vi "SEQ Destroy.vi"(8 "error in (no error)":errorcluster, 10 "wait for activity?":bool, 11 "Data Refnum":T1) -> (0 "error out":errorcluster, 3 "Final Data":T2)   [LabVIEW 2009]
doc: "This is a template VI for the SEQ Destroy functionality.\n\nAAL 9/09"
uses:
  Controls/SEQ Data.ctl
  Controls/SEQ DataRef.ctl
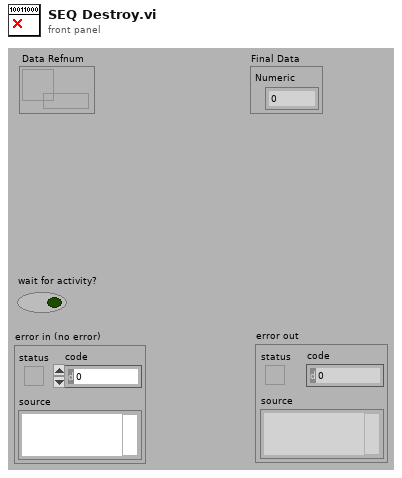
[diagram p1: front panel]
types:
  T1 = typedef "SEQ DataRef.ctl" = refnum<queue>
  T2 = typedef "SEQ Data.ctl" = cluster{"Numeric":dbl}
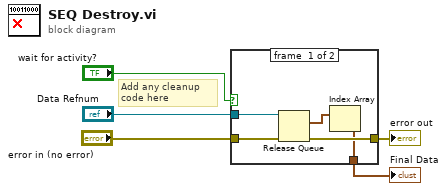
[diagram p0: block diagram]
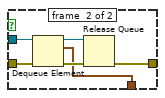
[diagram p2: hidden frame]
diagram:
  # "Add any cleanup\ncode here"
  n1 = case shown="False" "wait for activity?" {
    tunnel: "error in (no error)" -> [w8 w16]
    tunnel: "Data Refnum" -> [w7 w15]
    tunnel: [w10 w12] -> w3
    tunnel: [w6 w11] -> w2
    frame #0 {
      n2 = Release Queue(queue=w7, error in (no error)=w8) -> (remaining elements=w9:T2[], error out=w10:errorcluster)  [unwired: 2 out]
      n3 = Index Array(array=w9) -> (element=w6:T2)  [unwired: 1 in]
    }
    frame #1 {
      n4 = Dequeue Element(queue=w15, error in (no error)=w16) -> (queue out=w13:T1, element=w11:T2, error out=w14:errorcluster)  [unwired: 2 out]
      n5 = Release Queue(queue=w13, error in (no error)=w14) -> (error out=w12:errorcluster)  [unwired: 3 out]
    }
  }
  "Final Data" <- w2
  "error out" <- w3
